vi "DSF.Engine.Framework.Encapsulate Buffer.vi"(8 "error in (no error)":errorcluster, 10 "Buffer":refnum<class "DSF.Engine.Pointer.DBL.lvclass">, 11 "Framework in":refnum<class "DSF.Engine.Framework.lvclass">) -> (0 "error out":errorcluster, 2 "encapsulated Buffer":refnum<class "DSF.Engine.Pointer.DBL.lvclass">, 3 "Framework out":refnum<class "DSF.Engine.Framework.lvclass">)   [LabVIEW 2017, in "DSF.Engine.lvlib" / "DSF.Engine.Framework.lvclass"]
uses:
  DSF.Engine.Framework.lvclass
  Pointer/DSF.Engine.Pointer.DBL.lvclass
  C:/Program Files (x86)/National Instruments/LabVIEW 2017/vi.lib/National Instruments/Memory Manager/Classes/Pointer/Memory.Pointer.lvclass
  <vilib>/National Instruments/Memory Manager/Classes/Pointer/Memory.Pointer.lvclass/Memory.Pointer.ctl
  <vilib>/National Instruments/Memory Manager/Classes/Pointer/Memory.Pointer.Set Size.vi
  <vilib>/National Instruments/Memory Manager/Classes/Pointer/Memory.Pointer.Set Address.vi
  <vilib>/National Instruments/Memory Manager/Classes/Pointer/Memory.Pointer.Parameter Check.Null Pointer.vi
  <vilib>/National Instruments/Memory Manager/Classes/Pointer/Memory.Pointer.Set Allocated.vi
  <vilib>/National Instruments/Memory Manager/Classes/Pointer/Memory.Pointer.Errors.vi
  <vilib>/National Instruments/Memory Manager/Classes/Pointer/Memory.Pointer.Errors.Null Pointer.vi
  <vilib>/National Instruments/Memory Manager/Classes/Pointer/Memory.Pointer.Errors.Create Error.vi
  <vilib>/NI/Static Error Handling/VIs/Static Error Handling.Error Cluster Constant.vi
  <vilib>/NI/Static Error Handling/VIs/Static Error Handling.Error Cluster Constant (512B).vi
  <vilib>/NI/Static Error Handling/VIs/Static Error Handling.Parameters.Status.Set.vi
  <vilib>/NI/Static Error Handling/VIs/Static Error Handling.Parameters.Code.Set.vi
  <vilib>/NI/Static Error Handling/VIs/Static Error Handling.Parameters.VI Source.Set.vi
  <vilib>/National Instruments/Memory Manager/Constants/Memory.Constants.vi
  <vilib>/National Instruments/Memory Manager/Constants/Memory.Constants.Library Name.vi
  <vilib>/National Instruments/Memory Manager/Classes/Pointer/Memory.Pointer.Errors.Get Info.vi
  <vilib>/NI/Static Error Handling/VIs/Static Error Handling.Source Buffer.Write.String.vi
  <vilib>/National Instruments/Memory Manager/Classes/Pointer/Memory.Pointer.lvclass
panel:
  in  "size":u64 format="%d bytes"
  in  "address":u64 format="%016x"
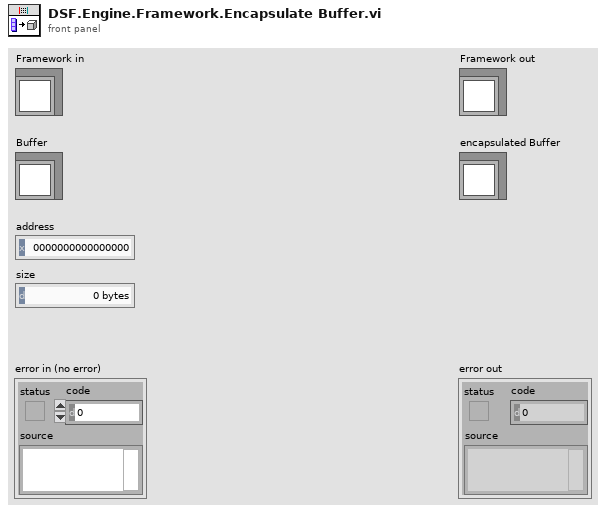
[diagram p1: front panel]
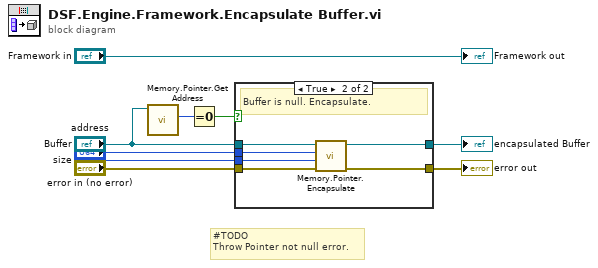
[diagram p0: block diagram]
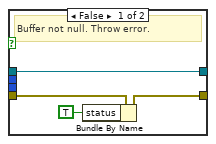
[diagram p2: hidden frame]
diagram:
  # "#TODO\nThrow Pointer not null error."
  n1 = call <vilib>:"Memory.Pointer.Get Address.vi"("Pointer in"="Buffer") -> ("address"=w9:u64)  [unwired: 9 in, 1 out]
  n2 = Equal To 0?(x=w9) -> (x = 0?=w1:bool)
  n3 = case shown="True" w1 {
    tunnel: "error in (no error)" -> [w13 w19]
    tunnel: [w12 w18] -> w6
    tunnel: "Buffer" -> [w10 w17]
    tunnel: [w10 w16] -> w4
    tunnel: "address" -> [_ w15]
    tunnel: "size" -> [_ w14]
    frame False {
      # "Buffer not null. Throw error."
      n4 = Bundle By Name(cluster=w13, "status"=TRUE) -> (w12:errorcluster)
    }
    frame True {
      # "Buffer is null. Encapsulate."
      n5 = call <vilib>:"Memory.Pointer.Encapsulate.vi"("error in (no error)"=w19, "size"=w14, "address"=w15, "Pointer type"=w17) -> ("error out"=w18:errorcluster, "Pointer out"=w16:refnum<class "DSF.Engine.Pointer.DBL.lvclass">)  [unwired: 6 in]
    }
  }
  "error out" <- w6
  "encapsulated Buffer" <- w4
  "Framework out" <- "Framework in"
